vi "P541.vi"(4 "Special Function In":string, 6 "Velocity":dbl, 7 "Abort":refnum<vi>, 8 "Axis":bool[](array[boolean]), 9 "Positions":dbl[](array[numeric]), 10 "Action":T1=enum."MVR", 11 "VISA In":refnum<visa-resource-name>) -> (0 "Special Function Out":string, 1 "Status":bool, 2 "Position Out":dbl[](array[numeric]), 3 "VISA Out":refnum<visa-resource-name>)   [LabVIEW 2011]
uses:
  Controls/StageStates.ctl
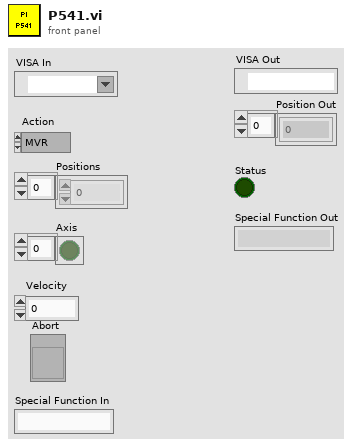
[diagram p1: front panel]
types:
  T1 = typedef "StageStates.ctl" = enum16{"POSITION", "MVR", "MOVE", "HALT", "ONTARGET", "ERROR", "EXIT", "HOME", "ZEROPOS", "NANOPOS", "QUIT", "ANALOG"}
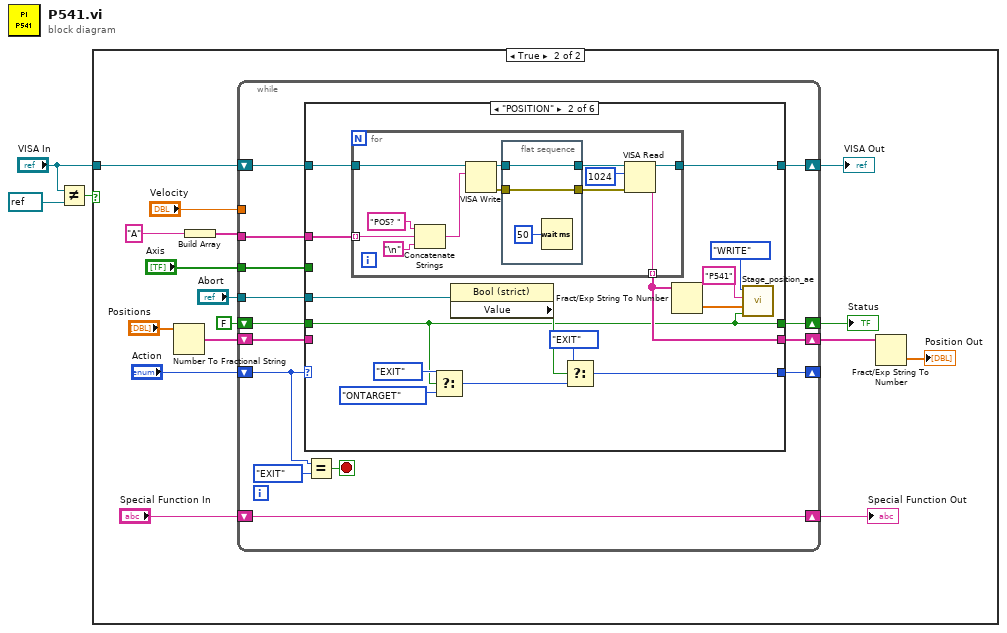
[diagram p0: block diagram]
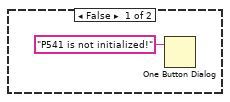
[diagram p2: hidden frame]
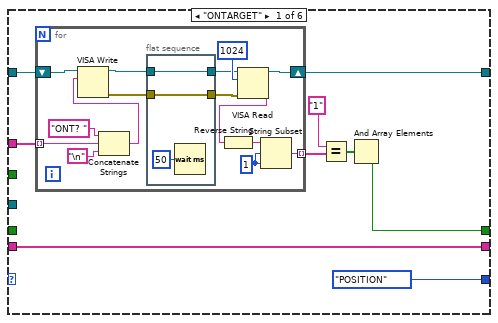
[diagram p3: hidden frame]
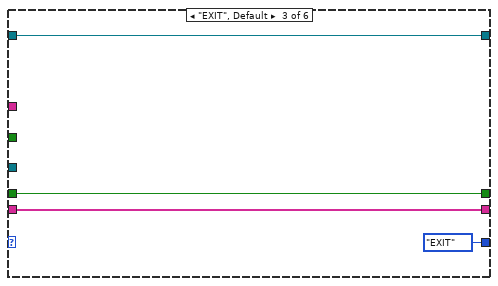
[diagram p4: hidden frame]
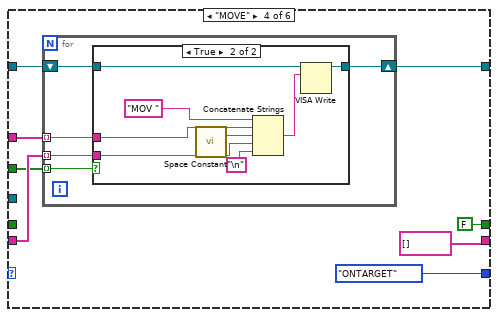
[diagram p5: hidden frame]
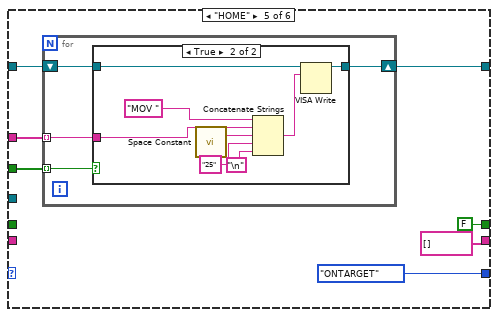
[diagram p7: hidden frame]
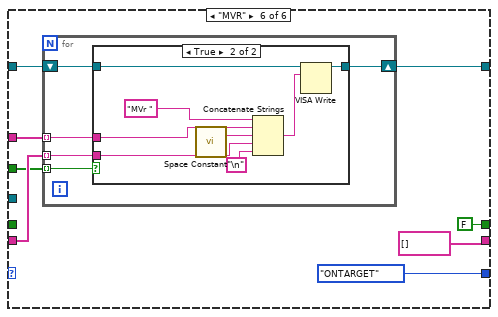
[diagram p9: hidden frame]
diagram:
  n1 = Not Equal?(x="VISA In", y=refnum<visa-resource-name> refnum ("VISA In")) -> (x != y?=w1:bool)
  n2 = case shown="True" w1 {
    tunnel: "VISA In" -> [_ w20]
    frame False {
      n3 = One Button Dialog(message="P541 is not initialized!") -> ()  [unwired: 1 in, 1 out]
    }
    frame True {
      n4 = Number To Fractional String(number="Positions") -> (F-format string=w10:string[])  [unwired: 3 in]
      n5 = Build Array("A") -> (w15:string[])
      n6 = while {
        tunnel: w15 -> [w34]
        shift-right: [w24] -> _
        shift-left: "Action" -> [w28]
        shift-right: [w31] -> w9
        shift-left: w10 -> [w32]
        shift-right: [w29] -> w18
        shift-left: FALSE -> [w30]
        tunnel: "Axis" -> [w27]
        shift-right: [w25] -> w12
        shift-left: "Special Function In" -> [w25]
        tunnel: "Velocity" -> [_]
        shift-right: [w23] -> w6
        shift-left: w20 -> [w33]
        tunnel: "Abort" -> [w21]
        stop <- w22 stop-if-true
        n7 = case shown="\"POSITION\"" w28 {
          tunnel: w34 -> [w43 w76 _ w103 w124 w145]
          tunnel: w33 -> [w37 w75 w95 w102 w123 w144]
          tunnel: w32 -> [w39 _ w93 w101 _ w143]
          tunnel: [w39 w65 w93 string[] [] string[] [] string[] []] -> w31
          tunnel: w30 -> [_ w62 w94 _ _ _]
          tunnel: [w38 w62 w94 FALSE FALSE FALSE] -> w29
          tunnel: w27 -> [_ _ _ w100 w122 w142]
          tunnel: [StageStates."POSITION" ("Action") w69 StageStates."EXIT" ("Action") StageStates."ONTARGET" ("Action") StageStates."ONTARGET" ("Action") StageStates."ONTARGET" ("Action")] -> w24
          tunnel: [w36 w74 w95 w98 w120 w140] -> w23
          tunnel: w21 -> [_ w63 _ _ _ _]
          frame "ONTARGET" {
            n8 = for {
              tunnel: w43 -> [w58] mode=indexing
              tunnel: [w57] -> w42 mode=indexing
              shift-right: [w48] -> w36
              shift-left: w37 -> [w49]
              w52 = 1 ("length (rest)")
              n9 = Concatenate Strings("ONT? " ("string"), w58, "\n") -> (w51:string)
              n10 = VISA Write(VISA resource name=w49, write buffer=w51) -> (VISA resource name out=w46:refnum<visa-resource-name>, error out=w44:errorcluster)  [unwired: 1 in, 1 out]
              n11 = flat-sequence {
                tunnel: [w61] -> w47
                tunnel: w46 -> [w61]
                tunnel: [w60] -> w45
                tunnel: w44 -> [w60]
                frame #0 {
                  n12 = Wait (ms)(milliseconds to wait=u32 50) -> ()  [unwired: 1 out]
                }
              }
              n13 = VISA Read(VISA resource name=w47, byte count=u32 1024, error in (no error)=w45) -> (VISA resource name out=w48:refnum<visa-resource-name>, read buffer=w50:string)  [unwired: 2 out]
              n14 = Reverse String(1:w50) -> (0:w53:string)
              n15 = String Subset(string=w53, offset (0)=w52, length (rest)=w52) -> (substring=w57:string)
            }
            n16 = Equal?(x="1", y=w42) -> (x = y?=w40:bool[])
            n17 = And Array Elements(Boolean array=w40) -> (logical AND=w38:bool)
          }
          frame "POSITION" {
            n18 = for {
              tunnel: w76 -> [w88] mode=indexing
              tunnel: w75 -> [w83]
              tunnel: [w82] -> w65 mode=indexing
              tunnel: [w77] -> w74
              n19 = Concatenate Strings("POS? " ("string"), w88, "\n") -> (w84:string)
              n20 = VISA Write(VISA resource name=w83, write buffer=w84) -> (VISA resource name out=w80:refnum<visa-resource-name>, error out=w78:errorcluster)  [unwired: 1 in, 1 out]
              n21 = flat-sequence {
                tunnel: [w91] -> w81
                tunnel: w80 -> [w91]
                tunnel: [w90] -> w79
                tunnel: w78 -> [w90]
                frame #0 {
                  n22 = Wait (ms)(milliseconds to wait=u32 50) -> ()  [unwired: 1 out]
                }
              }
              n23 = VISA Read(VISA resource name=w81, byte count=u32 1024, error in (no error)=w79) -> (VISA resource name out=w77:refnum<visa-resource-name>, read buffer=w82:string)  [unwired: 2 out]
            }
            n24 = Select(t=StageStates."EXIT" ("Action"), s=w62, f=StageStates."ONTARGET" ("Action")) -> (s? t:f=w72:T1)
            n25 = property class="Bool (strict)"(reference=w63) -> ("Value"=w64:bool)  [unwired: 1 in, 2 out]
            n26 = Select(t=StageStates."EXIT", s=w64, f=w72) -> (s? t:f=w69:T1)
            n27 = Fract/Exp String To Number(string=w65) -> (number=w68:dbl[])  [unwired: 3 in, 1 out]
            n28 = call "Stage_position_ae.vi"("Status In"=w62, "Position In"=w68, "StageID"="P541", "Enum"=enum16{"WRITE", "READ"}."WRITE") -> ()  [unwired: 6 in, 2 out]
          }
          frame "EXIT", Default {
          }
          frame "MOVE" {
            n29 = for {
              tunnel: w103 -> [w108] mode=indexing
              tunnel: w101 -> [w107] mode=indexing
              shift-right: [w105] -> w98
              shift-left: w102 -> [w106]
              tunnel: w100 -> [w104] mode=indexing
              n30 = case shown="True" w104 {
                tunnel: w108 -> [_ w115]
                tunnel: w107 -> [_ w112]
                tunnel: w106 -> [w109 w111]
                tunnel: [w109 w110] -> w105
                frame False {
                }
                frame True {
                  n31 = call <vilib>:"Space Constant.vi"() -> ("String"=w113:string)
                  n32 = Concatenate Strings("MOV ", w115, w113, w112, "\n") -> (w117:string)
                  n33 = VISA Write(VISA resource name=w111, write buffer=w117) -> (VISA resource name out=w110:refnum<visa-resource-name>)  [unwired: 1 in, 2 out]
                }
              }
            }
          }
          frame "HOME" {
            n34 = for {
              tunnel: w124 -> [w128] mode=indexing
              shift-right: [w126] -> w120
              shift-left: w123 -> [w127]
              tunnel: w122 -> [w125] mode=indexing
              n35 = case shown="True" w125 {
                tunnel: w128 -> [_ w135]
                tunnel: w127 -> [w129 w132]
                tunnel: [w129 w131] -> w126
                frame False {
                }
                frame True {
                  n36 = call <vilib>:"Space Constant.vi"() -> ("String"=w133:string)
                  n37 = Concatenate Strings("MOV ", w135, w133, "25" ("string"), "\n") -> (w137:string)
                  n38 = VISA Write(VISA resource name=w132, write buffer=w137) -> (VISA resource name out=w131:refnum<visa-resource-name>)  [unwired: 1 in, 2 out]
                }
              }
            }
          }
          frame "MVR" {
            n39 = for {
              tunnel: w145 -> [w150] mode=indexing
              tunnel: w143 -> [w149] mode=indexing
              shift-right: [w147] -> w140
              shift-left: w144 -> [w148]
              tunnel: w142 -> [w146] mode=indexing
              n40 = case shown="True" w146 {
                tunnel: w150 -> [_ w157]
                tunnel: w149 -> [_ w154]
                tunnel: w148 -> [w151 w153]
                tunnel: [w151 w152] -> w147
                frame False {
                }
                frame True {
                  n41 = call <vilib>:"Space Constant.vi"() -> ("String"=w155:string)
                  n42 = Concatenate Strings("MVr ", w157, w155, w154, "\n") -> (w159:string)
                  n43 = VISA Write(VISA resource name=w153, write buffer=w159) -> (VISA resource name out=w152:refnum<visa-resource-name>)  [unwired: 1 in, 2 out]
                }
              }
            }
          }
        }
        n44 = Equal?(x=w28, y=StageStates."EXIT") -> (x = y?=w22:bool)
      }
      "Status" <- w18
      "Special Function Out" <- w12
      "VISA Out" <- w6
      n45 = Fract/Exp String To Number(string=w9) -> (number=→"Position Out":dbl[])  [unwired: 3 in, 1 out]
    }
  }
